vi "SetLimiter.vi"(8 "error in":T7, 11 "Limiter Cluster":T1={"Limit"=FALSE, "Source"=-2147483648, "Value a.u."=-inf, "Sign"=-2147483648, "Loop"=FALSE, "Mode"=0} {"Mode" items=["Spectroscopy 1", "Spectroscopy 2", "Spectroscopy 3", "Calibration"]; "Sign" items=["[read only]"=-2147483648, "Source > Value"=0, "Source < Value"=1]; "Source" items=["[read only]"=-2147483648, "ADC 1"=0, "ADC 2"=1, "ADC 3"=2, "ADC 4"=3, "ADC 5"=4, "ADC 6"=5, "HF 1 Out"=7, "HF 1 df"=8, "SPM Z Out"=9, "HF 1"=12, "HF 1 Ampl"=13, "HF 1 Phase"=14, "LF LockIn Ampl"=16, "LF LockIn Phase"=17, "SPM Z Out inv"=18, "Counter"=23, "Crosslink 1"=29, "Crosslink 2"=30, "Pos X"=31, "Pos Y"=32]}) -> (0 "error out":T7, 3 "Output Cluster":T1={"Limit"=FALSE, "Source"=-2147483648, "Value a.u."=-inf, "Sign"=-2147483648, "Loop"=FALSE, "Mode"=0} {"Mode" items=["Spectroscopy 1", "Spectroscopy 2", "Spectroscopy 3", "Calibration"]; "Sign" items=["[read only]"=-2147483648, "Source > Value"=0, "Source < Value"=1]; "Source" items=["[read only]"=-2147483648, "ADC 1"=0, "ADC 2"=1, "ADC 3"=2, "ADC 4"=3, "ADC 5"=4, "ADC 6"=5, "HF 1 Out"=7, "HF 1 df"=8, "SPM Z Out"=9, "HF 1"=12, "HF 1 Ampl"=13, "HF 1 Phase"=14, "LF LockIn Ampl"=16, "LF LockIn Phase"=17, "SPM Z Out inv"=18, "Counter"=23, "Crosslink 1"=29, "Crosslink 2"=30, "Pos X"=31, "Pos Y"=32]})   [LabVIEW 2016]
doc: "This VI configures the limiter for any spectroscopy and activates it, if this is requested. The limiter cluster contains the following parameters:\n\n- Mode (integer) [0-2 -- Spectroscopy1-3]\n- Active (integer) [0 -- off; 1 -- on]\n- Source (integer) [0-5 -- ADC1-6; 6 -- SPM Z out; 7 -- SPM Z out inv; 8 -- AFM Signal; 9 -- AFM df; 10 -- AFM Aexc; 11 -- AFM Aosc; 12 -- AFM Phase; 13 -- LockIn Ampl; 14 -- LockIn Phase]\n- Sign (integer) [0 -- Source > Value; 1-- Source < Value]\nBy passing -Inf (float) or -2147483648 (integer) as input values, the corresponding parameter(s) will be read out."
uses:
  Controls/Limiter_Parameters.ctl
  Controls/Limiter-Active_Selection.ctl
  Controls/Limiter-Source_Selection.ctl
  Controls/Limiter-Sign_Selection.ctl
  Controls/Spectroscopy-loop_Selection.ctl
  Controls/Spectroscopy-Mode_Selection.ctl
  Controls/Error_Out.ctl
  Files_ASC500/DLL/ASC500_RemoteControlV27.dll
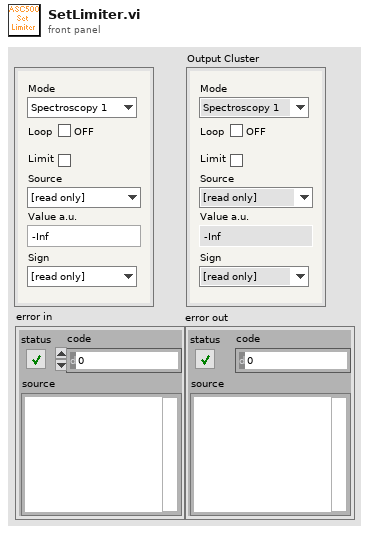
[diagram p1: front panel]
types:
  T1 = typedef "Limiter_Parameters.ctl" = cluster{"Limit":T2, "Source":T3, "Value a.u.":sgl, "Sign":T4, "Loop":T5, "Mode":T6}
  T2 = typedef "Limiter-Active_Selection.ctl" = bool
  T3 = typedef "Limiter-Source_Selection.ctl" = i32
  T4 = typedef "Limiter-Sign_Selection.ctl" = i32
  T5 = typedef "Spectroscopy-loop_Selection.ctl" = bool
  T6 = typedef "Spectroscopy-Mode_Selection.ctl" = u16
  T7 = typedef "Error_Out.ctl" = errorcluster
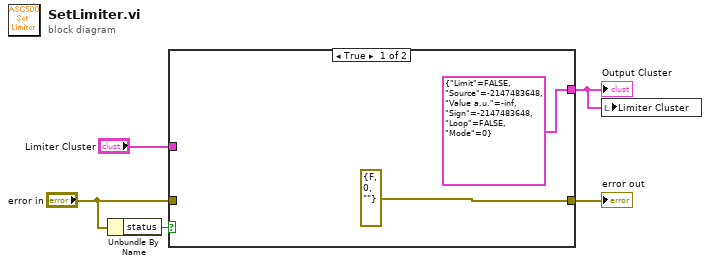
[diagram p0: block diagram]
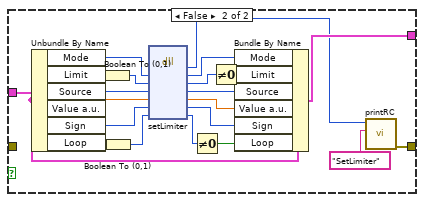
[diagram p2: hidden frame]
diagram:
  n1 = Unbundle By Name("error in") -> ("status"=w5:bool)
  n2 = case shown="True" w5 {
    tunnel: [T7 {"status"=FALSE, "code"=0, "source"=""} ("error out") w18] -> w4
    tunnel: "Limiter Cluster" -> [_ w20]
    tunnel: [T1 {"Limit"=FALSE, "Source"=-2147483648, "Value a.u."=-inf, "Sign"=-2147483648, "Loop"=FALSE, "Mode"=0} ("Limiter Cluster") w19] -> w1
    tunnel: "error in" -> [_ _]
    frame True {
    }
    frame False {
      n3 = Unbundle By Name(w20) -> ("Mode"=w28:T6, "Limit"=w15:T2, "Source"=w27:T3, "Value a.u."=w26:sgl, "Sign"=w25:T4, "Loop"=w11:T5)
      n4 = Boolean To (0,1)(Boolean=w15) -> (0, 1=w14:i16)
      n5 = Boolean To (0,1)(Boolean=w11) -> (0, 1=w10:i16)
      n6 = dll-call lib="G:/SCMOperations/Share/ELE/Produkt Information/ASC500/04 Remote Control/02 development versions/2018Nov06/Files_ASC500/DLL/ASC500_RemoteControlV27.dll" fn="setLimiter"("Mode"=w28, "Active"=w14, "Source"=w27, "Value"=w26, "Sign"=w25, "loop"=w10) -> ("return type"=w17:i32, "Mode"=w24:i32, "Active"=w12:i32, "Source"=w23:i32, "Value"=w22:sgl, "Sign"=w21:i32, "loop"=w9:i32)  [unwired: 3 in, 2 out]
      n7 = Not Equal To 0?(x=w9) -> (x != 0?=w8:bool)
      n8 = Not Equal To 0?(x=w12) -> (x != 0?=w13:bool)
      n9 = Bundle By Name(cluster=w20, "Mode"=w24, "Limit"=w13, "Source"=w23, "Value a.u."=w22, "Sign"=w21, "Loop"=w8) -> (w19:T1)
      n10 = call "printRC.vi"("additional information"="SetLimiter", "RC"=w17) -> ("error out"=w18:T7)  [unwired: 9 in]
    }
  }
  "error out" <- w4
  "Output Cluster" <- w1
  n11 = local write "Limiter Cluster"(w1) -> ()
